vi "S4GUI.vi"(7 "Tab ObsEng":enum32{"Obs", "CCD modes", "Guider", "Eng"}(tab)) -> ()   [LabVIEW 2018] (continued)
                n2889 = call "Write Exposure Time.vi"("error in (no error)"=w6491, "Exposure Time"=w6493, "Interface in"=w6494) -> ("error out"=w6490:errorcluster, "Interface out"=w6489:refnum<class "Interface.lvclass">)  [unwired: 7 in]
              }
            }
            n2890 = case shown="True" w6212 {
              tunnel: w6214 -> [w6501 w6512]
              tunnel: [w6501 w6502] -> w6218
              tunnel: w6213 -> [w6500 w6510]
              tunnel: [w6500 w6503] -> w6217
              frame False {
              }
              frame True {
                n2891 = call-dynamic "Write restoreExpTime.vi"("error in (no error)"=w6510, "restoreExpTime"=FALSE, "Interface in"=w6512) -> ("error out"=w6509:errorcluster, "Interface out"=w6511:refnum<class "Interface.lvclass">)  [unwired: 7 in]
                n2892 = call-dynamic "Read prev ExpTime.vi"("error in (no error)"=w6509, "Interface in"=w6511) -> ("error out"=w6507:errorcluster, "prev ExpTime"=w6504:dbl, "Interface out"=w6505:refnum<class "Interface.lvclass">)  [unwired: 7 in]
                n2893 = property on="Exptime ch2" class="DigNum (strict)"(error in=w6507, "Value"=w6504) -> (error out=w6506:errorcluster)  [unwired: 1 in, 1 out]
                n2894 = call "Write Exposure Time.vi"("error in (no error)"=w6506, "Exposure Time"=w6504, "Interface in"=w6505) -> ("error out"=w6503:errorcluster, "Interface out"=w6502:refnum<class "Interface.lvclass">)  [unwired: 7 in]
              }
            }
            n2895 = case shown="True" w6265 {
              tunnel: [w6514 w6515] -> w6271
              tunnel: [w6513 w6516] -> w6270
              tunnel: w6267 -> [w6514 w6525]
              tunnel: w6266 -> [w6513 w6523]
              frame False {
              }
              frame True {
                n2896 = call-dynamic "Write restoreExpTime.vi"("error in (no error)"=w6523, "restoreExpTime"=FALSE, "Interface in"=w6525) -> ("error out"=w6522:errorcluster, "Interface out"=w6524:refnum<class "Interface.lvclass">)  [unwired: 7 in]
                n2897 = call-dynamic "Read prev ExpTime.vi"("error in (no error)"=w6522, "Interface in"=w6524) -> ("error out"=w6518:errorcluster, "prev ExpTime"=w6519:dbl, "Interface out"=w6520:refnum<class "Interface.lvclass">)  [unwired: 7 in]
                n2898 = property on="Exptime ch1" class="DigNum (strict)"(error in=w6518, "Value"=w6519) -> (error out=w6517:errorcluster)  [unwired: 1 in, 1 out]
                n2899 = call "Write Exposure Time.vi"("error in (no error)"=w6517, "Exposure Time"=w6519, "Interface in"=w6520) -> ("error out"=w6516:errorcluster, "Interface out"=w6515:refnum<class "Interface.lvclass">)  [unwired: 7 in]
              }
            }
            n2900 = call-dynamic "Read PREV_FT.vi"("error in (no error)"=w6112, "Interface in"=w6111) -> ("error out"=w6104:errorcluster, "PREV_FT"=w6113:bool, "Interface out"=w6102:refnum<class "Interface.lvclass">)  [unwired: 7 in]
            n2901 = call-dynamic "Read PREV_FT.vi"("error in (no error)"=w6217, "Interface in"=w6218) -> ("error out"=w6210:errorcluster, "PREV_FT"=w6219:bool, "Interface out"=w6208:refnum<class "Interface.lvclass">)  [unwired: 7 in]
            n2902 = call-dynamic "Read PREV_FT.vi"("error in (no error)"=w6270, "Interface in"=w6271) -> ("error out"=w6261:errorcluster, "PREV_FT"=w6272:bool, "Interface out"=w6256:refnum<class "Interface.lvclass">)  [unwired: 7 in]
            n2903 = call-dynamic "Read PREV_FT.vi"("error in (no error)"=w6164, "Interface in"=w6165) -> ("error out"=w6157:errorcluster, "PREV_FT"=w6166:bool, "Interface out"=w6155:refnum<class "Interface.lvclass">)  [unwired: 7 in]
            n2904 = call-dynamic "Read target cluster.vi"("error in (no error)"=w6104, "Channel in"=w6105) -> ("error out"=w6099:errorcluster, "target cluster"=w6103:T31, "Channel out"=w6101:refnum<class "Channel.lvclass">)  [unwired: 7 in]
            n2905 = Bundle By Name(cluster=w6103, "SHUTTER_MODE"=u8 2, "FRAME_TRANSFER"=w6113) -> (w6100:T31)
            n2906 = call-dynamic "Read target cluster.vi"("error in (no error)"=w6210, "Channel in"=w6211) -> ("error out"=w6205:errorcluster, "target cluster"=w6209:T31, "Channel out"=w6207:refnum<class "Channel.lvclass">)  [unwired: 7 in]
            n2907 = Bundle By Name(cluster=w6209, "SHUTTER_MODE"=u8 2, "FRAME_TRANSFER"=w6219) -> (w6206:T31)
            n2908 = call-dynamic "Read target cluster.vi"("error in (no error)"=w6157, "Channel in"=w6158) -> ("error out"=w6152:errorcluster, "target cluster"=w6156:T31, "Channel out"=w6154:refnum<class "Channel.lvclass">)  [unwired: 7 in]
            n2909 = Bundle By Name(cluster=w6156, "SHUTTER_MODE"=u8 2, "FRAME_TRANSFER"=w6166) -> (w6153:T31)
            n2910 = call-dynamic "Read target cluster.vi"("error in (no error)"=w6261, "Channel in"=w6264) -> ("error out"=w6260:errorcluster, "target cluster"=w6258:T31, "Channel out"=w6263:refnum<class "Channel.lvclass">)  [unwired: 7 in]
            n2911 = Bundle By Name(cluster=w6258, "SHUTTER_MODE"=u8 2, "FRAME_TRANSFER"=w6272) -> (w6257:T31)
            n2912 = call-dynamic "Write target cluster.vi"("error in (no error)"=w6260, "target cluster"=w6257, "Channel in"=w6263) -> ("error out"=w6259:errorcluster, "Channel out"=w6262:refnum<class "Channel.lvclass">)  [unwired: 7 in]
            n2913 = call-dynamic "Write target cluster.vi"("error in (no error)"=w6099, "target cluster"=w6100, "Channel in"=w6101) -> ("error out"=w6098:errorcluster, "Channel out"=w6097:refnum<class "Channel.lvclass">)  [unwired: 7 in]
            n2914 = call-dynamic "Write target cluster.vi"("error in (no error)"=w6205, "target cluster"=w6206, "Channel in"=w6207) -> ("error out"=w6204:errorcluster, "Channel out"=w6203:refnum<class "Channel.lvclass">)  [unwired: 7 in]
            n2915 = call-dynamic "Write target cluster.vi"("error in (no error)"=w6152, "target cluster"=w6153, "Channel in"=w6154) -> ("error out"=w6151:errorcluster, "Channel out"=w6150:refnum<class "Channel.lvclass">)  [unwired: 7 in]
            n2916 = Flatten To String(anything=w6257, error in (no error)=w6259) -> (data string=w6305:string, error out=w6304:errorcluster)  [unwired: 2 in, 1 out]
            n2917 = Flatten To String(anything=w6100, error in (no error)=w6098) -> (data string=w6146:string, error out=w6145:errorcluster)  [unwired: 2 in, 1 out]
            n2918 = Flatten To String(anything=w6206, error in (no error)=w6204) -> (data string=w6243:string, error out=w6244:errorcluster)  [unwired: 2 in, 1 out]
            n2919 = Flatten To String(anything=w6153, error in (no error)=w6151) -> (data string=w6190:string, error out=w6191:errorcluster)  [unwired: 2 in, 1 out]
            n2920 = call "Write flatted cluster.vi"("error in (no error)"=w6304, "flatted cluster"=w6305, "Interface in"=w6256) -> ("error out"=w6301:errorcluster, "Interface out"=w6302:refnum<class "Interface.lvclass">)  [unwired: 7 in]
            n2921 = call "Write flatted cluster.vi"("error in (no error)"=w6145, "flatted cluster"=w6146, "Interface in"=w6102) -> ("error out"=w6142:errorcluster, "Interface out"=w6143:refnum<class "Interface.lvclass">)  [unwired: 7 in]
            n2922 = call "Write flatted cluster.vi"("error in (no error)"=w6244, "flatted cluster"=w6243, "Interface in"=w6208) -> ("error out"=w6247:errorcluster, "Interface out"=w6246:refnum<class "Interface.lvclass">)  [unwired: 7 in]
            n2923 = call "Write flatted cluster.vi"("error in (no error)"=w6191, "flatted cluster"=w6190, "Interface in"=w6155) -> ("error out"=w6194:errorcluster, "Interface out"=w6193:refnum<class "Interface.lvclass">)  [unwired: 7 in]
            n2924 = call-dynamic "Write Interface.vi"("error in (no error)"=w6301, "Interface.lvclass"=w6302, "Channel in"=w6262) -> ("error out"=w6299:errorcluster, "Channel out"=w6298:refnum<class "Channel.lvclass">)  [unwired: 7 in]
            n2925 = call-dynamic "Write Interface.vi"("error in (no error)"=w6142, "Interface.lvclass"=w6143, "Channel in"=w6097) -> ("error out"=w6140:errorcluster, "Channel out"=w6139:refnum<class "Channel.lvclass">)  [unwired: 7 in]
            n2926 = call-dynamic "Write Interface.vi"("error in (no error)"=w6247, "Interface.lvclass"=w6246, "Channel in"=w6203) -> ("error out"=w6249:errorcluster, "Channel out"=w6250:refnum<class "Channel.lvclass">)  [unwired: 7 in]
            n2927 = call-dynamic "Write Interface.vi"("error in (no error)"=w6194, "Interface.lvclass"=w6193, "Channel in"=w6150) -> ("error out"=w6196:errorcluster, "Channel out"=w6197:refnum<class "Channel.lvclass">)  [unwired: 7 in]
            n2928 = call "Write section_name.vi"("error in (no error)"=w6299, "section_name"="CCD_ACS1", "Channel in"=w6298) -> ("error out"=w6300:errorcluster, "Channel out"=w6295:refnum<class "Channel.lvclass">)  [unwired: 7 in]
            n2929 = call "Write section_name.vi"("error in (no error)"=w6140, "section_name"="CCD_ACS4", "Channel in"=w6139) -> ("error out"=w6141:errorcluster, "Channel out"=w6136:refnum<class "Channel.lvclass">)  [unwired: 7 in]
            n2930 = call "Write section_name.vi"("error in (no error)"=w6249, "section_name"="CCD_ACS2", "Channel in"=w6250) -> ("error out"=w6248:errorcluster, "Channel out"=w6253:refnum<class "Channel.lvclass">)  [unwired: 7 in]
            n2931 = call "Write section_name.vi"("error in (no error)"=w6196, "section_name"="CCD_ACS3", "Channel in"=w6197) -> ("error out"=w6195:errorcluster, "Channel out"=w6200:refnum<class "Channel.lvclass">)  [unwired: 7 in]
            n2932 = call-dynamic "save config.vi"("error in (no error)"=w6300, "file config"="lastsaved.cfg", "Channel in"=w6295) -> ("error out"=w6275:errorcluster, "Channel out"=w6276:refnum<class "Channel.lvclass">)  [unwired: 7 in]
            n2933 = call-dynamic "save config.vi"("error in (no error)"=w6141, "file config"="lastsaved.cfg", "Channel in"=w6136) -> ("error out"=w6116:errorcluster, "Channel out"=w6117:refnum<class "Channel.lvclass">)  [unwired: 7 in]
            n2934 = call-dynamic "save config.vi"("error in (no error)"=w6248, "file config"="lastsaved.cfg", "Channel in"=w6253) -> ("error out"=w6222:errorcluster, "Channel out"=w6223:refnum<class "Channel.lvclass">)  [unwired: 7 in]
            n2935 = call-dynamic "save config.vi"("error in (no error)"=w6195, "file config"="lastsaved.cfg", "Channel in"=w6200) -> ("error out"=w6169:errorcluster, "Channel out"=w6170:refnum<class "Channel.lvclass">)  [unwired: 7 in]
            n2936 = local read "Filter1"() -> (w6277:u8)
            n2937 = local read "Filter2"() -> (w6224:u8)
            n2938 = local read "Filter4"() -> (w6118:u8)
            n2939 = local read "Filter3"() -> (w6171:u8)
            n2940 = call-dynamic "Write Filter.vi"("error in (no error)"=w6275, "Filter"=w6277, "Channel in"=w6276) -> ("error out"=w6284:errorcluster, "Channel out"=w6285:refnum<class "Channel.lvclass">)  [unwired: 7 in]
            n2941 = call-dynamic "Write Filter.vi"("error in (no error)"=w6169, "Filter"=w6171, "Channel in"=w6170) -> ("error out"=w6178:errorcluster, "Channel out"=w6179:refnum<class "Channel.lvclass">)  [unwired: 7 in]
            n2942 = call-dynamic "Write Filter.vi"("error in (no error)"=w6222, "Filter"=w6224, "Channel in"=w6223) -> ("error out"=w6231:errorcluster, "Channel out"=w6232:refnum<class "Channel.lvclass">)  [unwired: 7 in]
            n2943 = call-dynamic "Write Filter.vi"("error in (no error)"=w6116, "Filter"=w6118, "Channel in"=w6117) -> ("error out"=w6125:errorcluster, "Channel out"=w6126:refnum<class "Channel.lvclass">)  [unwired: 7 in]
            n2944 = call-dynamic "Read Interface.vi"("error in (no error)"=w6231, "Channel in"=w6232) -> ("error out"=w6229:errorcluster, "Interface.lvclass"=w6234:refnum<class "Interface.lvclass">, "Channel out"=w6233:refnum<class "Channel.lvclass">)  [unwired: 7 in]
            n2945 = call-dynamic "Read Interface.vi"("error in (no error)"=w6178, "Channel in"=w6179) -> ("error out"=w6176:errorcluster, "Interface.lvclass"=w6181:refnum<class "Interface.lvclass">, "Channel out"=w6180:refnum<class "Channel.lvclass">)  [unwired: 7 in]
            n2946 = call-dynamic "Read Interface.vi"("error in (no error)"=w6284, "Channel in"=w6285) -> ("error out"=w6282:errorcluster, "Interface.lvclass"=w6287:refnum<class "Interface.lvclass">, "Channel out"=w6286:refnum<class "Channel.lvclass">)  [unwired: 7 in]
            n2947 = call-dynamic "Read Interface.vi"("error in (no error)"=w6125, "Channel in"=w6126) -> ("error out"=w6123:errorcluster, "Interface.lvclass"=w6128:refnum<class "Interface.lvclass">, "Channel out"=w6127:refnum<class "Channel.lvclass">)  [unwired: 7 in]
            n2948 = call-dynamic "Write Suffix.vi"("error in (no error)"=w6282, "Suffix"=w6310, "Interface in"=w6287) -> ("error out"=w6278:errorcluster, "Interface out"=w6288:refnum<class "Interface.lvclass">)  [unwired: 7 in]
            n2949 = call-dynamic "Write Suffix.vi"("error in (no error)"=w6229, "Suffix"=w6310, "Interface in"=w6234) -> ("error out"=w6225:errorcluster, "Interface out"=w6235:refnum<class "Interface.lvclass">)  [unwired: 7 in]
            n2950 = call-dynamic "Write Suffix.vi"("error in (no error)"=w6176, "Suffix"=w6310, "Interface in"=w6181) -> ("error out"=w6172:errorcluster, "Interface out"=w6182:refnum<class "Interface.lvclass">)  [unwired: 7 in]
            n2951 = call-dynamic "Write Suffix.vi"("error in (no error)"=w6123, "Suffix"=w6310, "Interface in"=w6128) -> ("error out"=w6119:errorcluster, "Interface out"=w6129:refnum<class "Interface.lvclass">)  [unwired: 7 in]
            n2952 = call-dynamic "Write ObsType.vi"("error in (no error)"=w6225, "ObsType"=w6309, "Interface in"=w6235) -> ("error out"=w6226:errorcluster, "Interface out"=w6236:refnum<class "Interface.lvclass">)  [unwired: 7 in]
            n2953 = call-dynamic "Write ObsType.vi"("error in (no error)"=w6172, "ObsType"=w6309, "Interface in"=w6182) -> ("error out"=w6173:errorcluster, "Interface out"=w6183:refnum<class "Interface.lvclass">)  [unwired: 7 in]
            n2954 = call-dynamic "Write ObsType.vi"("error in (no error)"=w6278, "ObsType"=w6309, "Interface in"=w6288) -> ("error out"=w6279:errorcluster, "Interface out"=w6289:refnum<class "Interface.lvclass">)  [unwired: 7 in]
            n2955 = call-dynamic "Write ObsType.vi"("error in (no error)"=w6119, "ObsType"=w6309, "Interface in"=w6129) -> ("error out"=w6120:errorcluster, "Interface out"=w6130:refnum<class "Interface.lvclass">)  [unwired: 7 in]
            n2956 = call-dynamic "Write Object.vi"("error in (no error)"=w6226, "Object"=w6313, "Interface in"=w6236) -> ("error out"=w6227:errorcluster, "Interface out"=w6237:refnum<class "Interface.lvclass">)  [unwired: 7 in]
            n2957 = call-dynamic "Write Object.vi"("error in (no error)"=w6173, "Object"=w6313, "Interface in"=w6183) -> ("error out"=w6174:errorcluster, "Interface out"=w6184:refnum<class "Interface.lvclass">)  [unwired: 7 in]
            n2958 = call-dynamic "Write Object.vi"("error in (no error)"=w6279, "Object"=w6313, "Interface in"=w6289) -> ("error out"=w6280:errorcluster, "Interface out"=w6290:refnum<class "Interface.lvclass">)  [unwired: 7 in]
            n2959 = call-dynamic "Write Object.vi"("error in (no error)"=w6120, "Object"=w6313, "Interface in"=w6130) -> ("error out"=w6121:errorcluster, "Interface out"=w6131:refnum<class "Interface.lvclass">)  [unwired: 7 in]
            n2960 = call-dynamic "Write Comments.vi"("error in (no error)"=w6227, "Comments"=w6312, "Interface in"=w6237) -> ("error out"=w6228:errorcluster, "Interface out"=w6238:refnum<class "Interface.lvclass">)  [unwired: 7 in]
            n2961 = call-dynamic "Write Comments.vi"("error in (no error)"=w6174, "Comments"=w6312, "Interface in"=w6184) -> ("error out"=w6175:errorcluster, "Interface out"=w6185:refnum<class "Interface.lvclass">)  [unwired: 7 in]
            n2962 = call-dynamic "Write Comments.vi"("error in (no error)"=w6280, "Comments"=w6312, "Interface in"=w6290) -> ("error out"=w6281:errorcluster, "Interface out"=w6291:refnum<class "Interface.lvclass">)  [unwired: 7 in]
            n2963 = call-dynamic "Write Comments.vi"("error in (no error)"=w6121, "Comments"=w6312, "Interface in"=w6131) -> ("error out"=w6122:errorcluster, "Interface out"=w6132:refnum<class "Interface.lvclass">)  [unwired: 7 in]
            n2964 = call-dynamic "Write Observer.vi"("error in (no error)"=w6228, "Observer"=w6311, "Interface in"=w6238) -> ("error out"=w6230:errorcluster, "Interface out"=w6239:refnum<class "Interface.lvclass">)  [unwired: 7 in]
            n2965 = call-dynamic "Write Observer.vi"("error in (no error)"=w6175, "Observer"=w6311, "Interface in"=w6185) -> ("error out"=w6177:errorcluster, "Interface out"=w6186:refnum<class "Interface.lvclass">)  [unwired: 7 in]
            n2966 = call-dynamic "Write Observer.vi"("error in (no error)"=w6281, "Observer"=w6311, "Interface in"=w6291) -> ("error out"=w6283:errorcluster, "Interface out"=w6292:refnum<class "Interface.lvclass">)  [unwired: 7 in]
            n2967 = call-dynamic "Write Observer.vi"("error in (no error)"=w6122, "Observer"=w6311, "Interface in"=w6132) -> ("error out"=w6124:errorcluster, "Interface out"=w6133:refnum<class "Interface.lvclass">)  [unwired: 7 in]
            n2968 = call-dynamic "Write Interface.vi"("error in (no error)"=w6230, "Interface.lvclass"=w6239, "Channel in"=w6233) -> ("error out"=w6220:errorcluster, "Channel out"=w6221:refnum<class "Channel.lvclass">)  [unwired: 7 in]
            n2969 = call-dynamic "Write Interface.vi"("error in (no error)"=w6177, "Interface.lvclass"=w6186, "Channel in"=w6180) -> ("error out"=w6167:errorcluster, "Channel out"=w6168:refnum<class "Channel.lvclass">)  [unwired: 7 in]
            n2970 = call-dynamic "Write Interface.vi"("error in (no error)"=w6283, "Interface.lvclass"=w6292, "Channel in"=w6286) -> ("error out"=w6273:errorcluster, "Channel out"=w6274:refnum<class "Channel.lvclass">)  [unwired: 7 in]
            n2971 = call-dynamic "Write Interface.vi"("error in (no error)"=w6124, "Interface.lvclass"=w6133, "Channel in"=w6127) -> ("error out"=w6114:errorcluster, "Channel out"=w6115:refnum<class "Channel.lvclass">)  [unwired: 7 in]
            n2972 = case shown="True" w6096 {
              tunnel: [w6441 w6462] -> w6294
              tunnel: [w6440 w6461] -> w6293
              tunnel: w6274 -> [w6441 w6460]
              tunnel: w6273 -> [w6440 w6459]
              frame False {
              }
              frame True {
                # "command SET EXPTIME"
                # "command WRITE_SETUP"
                # "command SET SUFFIX"
                n2973 = call-dynamic "Read State Machine.vi"("error in (no error)"=w6459, "Device in"=w6460) -> ("error out"=w6449:errorcluster, "State Machine.lvclass"=w6451:refnum<class "State Machine.lvclass">, "Device out"=w6464:refnum<class "Channel.lvclass">)  [unwired: 7 in]
                n2974 = call-dynamic "Read ref StatesQueue.vi"("error in (no error)"=w6449, "State Machine in"=w6451) -> ("error out"=w6457:errorcluster, "ref StatesQueue"=w6447:refnum<queue>, "State Machine out"=w6458:refnum<class "State Machine.lvclass">)  [unwired: 7 in]
                n2975 = Flush Queue(queue=w6447, error in (no error)=w6457) -> (queue out=w6446:refnum<queue>, error out=w6454:errorcluster)  [unwired: 1 out]
                n2976 = Enqueue Element(queue=w6446, element=u32 300 ("State"), error in (no error)=w6454) -> (queue out=w6445:refnum<queue>, error out=w6444:errorcluster)  [unwired: 1 in, 1 out]
                n2977 = disable-structure shown="Enabled" {
                  disable-tunnel: w6445 -> [w6470 w6473]
                  disable-tunnel: w6444 -> [w6469 w6472]
                  disable-tunnel: [w6468 w6472] -> w6443
                  disable-tunnel: [w6467 w6473] -> w6442
                  frame Disabled {
                    n2978 = Enqueue Element(queue=w6470, element=u32 305 ("State"), error in (no error)=w6469) -> (queue out=w6467:refnum<queue>, error out=w6468:errorcluster)  [unwired: 1 in, 1 out]
                  }
                  frame Enabled {
                  }
                }
                n2979 = Enqueue Element(queue=w6442, element=u32 60 ("State"), error in (no error)=w6443) -> (queue out=w6456:refnum<queue>, error out=w6455:errorcluster)  [unwired: 1 in, 1 out]
                n2980 = call-dynamic "Write ref StatesQueue.vi"("error in (no error)"=w6455, "ref StatesQueue"=w6456, "State Machine in"=w6458) -> ("error out"=w6448:errorcluster, "State Machine out"=w6450:refnum<class "State Machine.lvclass">)  [unwired: 7 in]
                n2981 = call-dynamic "Write State.vi"("error in (no error)"=w6448, "State"=0, "State Machine in"=w6450) -> ("error out"=w6466:errorcluster, "State Machine out"=w6463:refnum<class "State Machine.lvclass">)  [unwired: 7 in]
                n2982 = call-dynamic "Write State Machine.vi"("error in (no error)"=w6466, "State Machine.lvclass"=w6463, "Device in"=w6464) -> ("error out"=w6461:errorcluster, "Device out"=w6462:refnum<class "Channel.lvclass">)  [unwired: 7 in]
              }
            }
            n2983 = case shown="True" w6095 {
              tunnel: [w6406 w6432] -> w6255
              tunnel: [w6407 w6431] -> w6254
              tunnel: w6221 -> [w6407 w6426]
              tunnel: w6220 -> [w6406 w6425]
              frame False {
              }
              frame True {
                # "command SET EXPTIME"
                # "command WRITE_SETUP"
                # "command SET SUFFIX"
                n2984 = call-dynamic "Read State Machine.vi"("error in (no error)"=w6425, "Device in"=w6426) -> ("error out"=w6416:errorcluster, "State Machine.lvclass"=w6417:refnum<class "State Machine.lvclass">, "Device out"=w6429:refnum<class "Channel.lvclass">)  [unwired: 7 in]
                n2985 = call-dynamic "Read ref StatesQueue.vi"("error in (no error)"=w6416, "State Machine in"=w6417) -> ("error out"=w6423:errorcluster, "ref StatesQueue"=w6415:refnum<queue>, "State Machine out"=w6424:refnum<class "State Machine.lvclass">)  [unwired: 7 in]
                n2986 = Flush Queue(queue=w6415, error in (no error)=w6423) -> (queue out=w6414:refnum<queue>, error out=w6420:errorcluster)  [unwired: 1 out]
                n2987 = Enqueue Element(queue=w6414, element=u32 300 ("State"), error in (no error)=w6420) -> (queue out=w6409:refnum<queue>, error out=w6411:errorcluster)  [unwired: 1 in, 1 out]
                n2988 = disable-structure shown="Enabled" {
                  disable-tunnel: w6411 -> [w6436 w6438]
                  disable-tunnel: [w6435 w6438] -> w6410
                  disable-tunnel: w6409 -> [w6434 w6439]
                  disable-tunnel: [w6433 w6439] -> w6408
                  frame Disabled {
                    n2989 = Enqueue Element(queue=w6434, element=u32 305 ("State"), error in (no error)=w6436) -> (queue out=w6433:refnum<queue>, error out=w6435:errorcluster)  [unwired: 1 in, 1 out]
                  }
                  frame Enabled {
                  }
                }
                n2990 = Enqueue Element(queue=w6408, element=u32 60 ("State"), error in (no error)=w6410) -> (queue out=w6422:refnum<queue>, error out=w6421:errorcluster)  [unwired: 1 in, 1 out]
                n2991 = call-dynamic "Write ref StatesQueue.vi"("error in (no error)"=w6421, "ref StatesQueue"=w6422, "State Machine in"=w6424) -> ("error out"=w6412:errorcluster, "State Machine out"=w6413:refnum<class "State Machine.lvclass">)  [unwired: 7 in]
                n2992 = call-dynamic "Write State.vi"("error in (no error)"=w6412, "State"=0, "State Machine in"=w6413) -> ("error out"=w6427:errorcluster, "State Machine out"=w6430:refnum<class "State Machine.lvclass">)  [unwired: 7 in]
                n2993 = call-dynamic "Write State Machine.vi"("error in (no error)"=w6427, "State Machine.lvclass"=w6430, "Device in"=w6429) -> ("error out"=w6432:errorcluster, "Device out"=w6431:refnum<class "Channel.lvclass">)  [unwired: 7 in]
              }
            }
            n2994 = case shown="True" w6094 {
              tunnel: [w6372 w6398] -> w6202
              tunnel: [w6373 w6397] -> w6201
              tunnel: w6168 -> [w6373 w6392]
              tunnel: w6167 -> [w6372 w6391]
              frame False {
              }
              frame True {
                # "command SET EXPTIME"
                # "command WRITE_SETUP"
                # "command SET SUFFIX"
                n2995 = call-dynamic "Read State Machine.vi"("error in (no error)"=w6391, "Device in"=w6392) -> ("error out"=w6381:errorcluster, "State Machine.lvclass"=w6380:refnum<class "State Machine.lvclass">, "Device out"=w6395:refnum<class "Channel.lvclass">)  [unwired: 7 in]
                n2996 = call-dynamic "Read ref StatesQueue.vi"("error in (no error)"=w6381, "State Machine in"=w6380) -> ("error out"=w6389:errorcluster, "ref StatesQueue"=w6383:refnum<queue>, "State Machine out"=w6390:refnum<class "State Machine.lvclass">)  [unwired: 7 in]
                n2997 = Flush Queue(queue=w6383, error in (no error)=w6389) -> (queue out=w6382:refnum<queue>, error out=w6386:errorcluster)  [unwired: 1 out]
                n2998 = Enqueue Element(queue=w6382, element=u32 300 ("State"), error in (no error)=w6386) -> (queue out=w6376:refnum<queue>, error out=w6377:errorcluster)  [unwired: 1 in, 1 out]
                n2999 = disable-structure shown="Enabled" {
                  disable-tunnel: w6377 -> [w6402 w6404]
                  disable-tunnel: w6376 -> [w6401 w6405]
                  disable-tunnel: [w6400 w6404] -> w6375
                  disable-tunnel: [w6399 w6405] -> w6374
                  frame Disabled {
                    n3000 = Enqueue Element(queue=w6401, element=u32 305 ("State"), error in (no error)=w6402) -> (queue out=w6399:refnum<queue>, error out=w6400:errorcluster)  [unwired: 1 in, 1 out]
                  }
                  frame Enabled {
                  }
                }
                n3001 = Enqueue Element(queue=w6374, element=u32 60 ("State"), error in (no error)=w6375) -> (queue out=w6388:refnum<queue>, error out=w6387:errorcluster)  [unwired: 1 in, 1 out]
                n3002 = call-dynamic "Write ref StatesQueue.vi"("error in (no error)"=w6387, "ref StatesQueue"=w6388, "State Machine in"=w6390) -> ("error out"=w6378:errorcluster, "State Machine out"=w6379:refnum<class "State Machine.lvclass">)  [unwired: 7 in]
                n3003 = call-dynamic "Write State.vi"("error in (no error)"=w6378, "State"=0, "State Machine in"=w6379) -> ("error out"=w6393:errorcluster, "State Machine out"=w6396:refnum<class "State Machine.lvclass">)  [unwired: 7 in]
                n3004 = call-dynamic "Write State Machine.vi"("error in (no error)"=w6393, "State Machine.lvclass"=w6396, "Device in"=w6395) -> ("error out"=w6398:errorcluster, "Device out"=w6397:refnum<class "Channel.lvclass">)  [unwired: 7 in]
              }
            }
            n3005 = case shown="True" w6093 {
              tunnel: [w6338 w6360] -> w6135
              tunnel: [w6339 w6359] -> w6134
              tunnel: w6115 -> [w6339 w6358]
              tunnel: w6114 -> [w6338 w6357]
              frame False {
              }
              frame True {
                # "command SET EXPTIME"
                # "command WRITE_SETUP"
                # "command SET SUFFIX"
                n3006 = call-dynamic "Read State Machine.vi"("error in (no error)"=w6357, "Device in"=w6358) -> ("error out"=w6346:errorcluster, "State Machine.lvclass"=w6347:refnum<class "State Machine.lvclass">, "Device out"=w6362:refnum<class "Channel.lvclass">)  [unwired: 7 in]
                n3007 = call-dynamic "Read ref StatesQueue.vi"("error in (no error)"=w6346, "State Machine in"=w6347) -> ("error out"=w6355:errorcluster, "ref StatesQueue"=w6349:refnum<queue>, "State Machine out"=w6356:refnum<class "State Machine.lvclass">)  [unwired: 7 in]
                n3008 = Flush Queue(queue=w6349, error in (no error)=w6355) -> (queue out=w6348:refnum<queue>, error out=w6352:errorcluster)  [unwired: 1 out]
                n3009 = Enqueue Element(queue=w6348, element=u32 300 ("State"), error in (no error)=w6352) -> (queue out=w6343:refnum<queue>, error out=w6341:errorcluster)  [unwired: 1 in, 1 out]
                n3010 = disable-structure shown="Enabled" {
                  disable-tunnel: w6343 -> [w6368 w6371]
                  disable-tunnel: [w6367 w6371] -> w6342
                  disable-tunnel: w6341 -> [w6366 w6370]
                  disable-tunnel: [w6365 w6370] -> w6340
                  frame Disabled {
                    n3011 = Enqueue Element(queue=w6368, element=u32 305 ("State"), error in (no error)=w6366) -> (queue out=w6367:refnum<queue>, error out=w6365:errorcluster)  [unwired: 1 in, 1 out]
                  }
                  frame Enabled {
                  }
                }
                n3012 = Enqueue Element(queue=w6342, element=u32 60 ("State"), error in (no error)=w6340) -> (queue out=w6354:refnum<queue>, error out=w6353:errorcluster)  [unwired: 1 in, 1 out]
                n3013 = call-dynamic "Write ref StatesQueue.vi"("error in (no error)"=w6353, "ref StatesQueue"=w6354, "State Machine in"=w6356) -> ("error out"=w6344:errorcluster, "State Machine out"=w6345:refnum<class "State Machine.lvclass">)  [unwired: 7 in]
                n3014 = call-dynamic "Write State.vi"("error in (no error)"=w6344, "State"=0, "State Machine in"=w6345) -> ("error out"=w6364:errorcluster, "State Machine out"=w6361:refnum<class "State Machine.lvclass">)  [unwired: 7 in]
                n3015 = call-dynamic "Write State Machine.vi"("error in (no error)"=w6364, "State Machine.lvclass"=w6361, "Device in"=w6362) -> ("error out"=w6360:errorcluster, "Device out"=w6359:refnum<class "Channel.lvclass">)  [unwired: 7 in]
              }
            }
            n3016 = call-dynamic "Write Channel.vi"("error in (no error)"=w6255, "Channel.lvclass"=w6254, "Acquisition in"=w6240) -> ("error out"=w6334:errorcluster, "Acquisition out"=w6335:refnum<class "Acquisition.lvclass">)  [unwired: 7 in]
            n3017 = call-dynamic "Write Channel.vi"("error in (no error)"=w6135, "Channel.lvclass"=w6134, "Acquisition in"=w6149) -> ("error out"=w6330:errorcluster, "Acquisition out"=w6331:refnum<class "Acquisition.lvclass">)  [unwired: 7 in]
            n3018 = call-dynamic "Write Channel.vi"("error in (no error)"=w6293, "Channel.lvclass"=w6294, "Acquisition in"=w6308) -> ("error out"=w6336:errorcluster, "Acquisition out"=w6337:refnum<class "Acquisition.lvclass">)  [unwired: 7 in]
            n3019 = call-dynamic "Write Channel.vi"("error in (no error)"=w6202, "Channel.lvclass"=w6201, "Acquisition in"=w6187) -> ("error out"=w6332:errorcluster, "Acquisition out"=w6333:refnum<class "Acquisition.lvclass">)  [unwired: 7 in]
          }
          frame "OBJECT", Default {
            # "20250918:\nACS corrigido,\nnão precisa restaurar\nExpTime. Causou bug\nquando ExpTime tinha\nvalor default (1E-5s)"
            # "nome do arquivo .cfg"
            # "seção no arquivo .cfg"
            # "open"
            # "nome do arquivo .cfg"
            # "seção no arquivo .cfg"
            # "open"
            # "nome do arquivo .cfg"
            # "seção no arquivo .cfg"
            # "open"
            # "nome do arquivo .cfg"
            # "seção no arquivo .cfg"
            # "open"
            # "OBJECT, DFLAT,SFLAT and FOCUS: Shutter automatically open and restore FRAME_TRANSFER."
            n3020 = call "Read connection.vi"("error in (no error)"=w6751, "Server in"=w6752) -> ("error out"=w6757:errorcluster, "connection"=w6527:bool, "Server out"=w6758:refnum<class "Acquisition.lvclass">)  [unwired: 7 in]
            n3021 = call "Read connection.vi"("error in (no error)"=w6749, "Server in"=w6750) -> ("error out"=w6755:errorcluster, "connection"=w6528:bool, "Server out"=w6756:refnum<class "Acquisition.lvclass">)  [unwired: 7 in]
            n3022 = call "Read connection.vi"("error in (no error)"=w6761, "Server in"=w6762) -> ("error out"=w6759:errorcluster, "connection"=w6526:bool, "Server out"=w6760:refnum<class "Acquisition.lvclass">)  [unwired: 7 in]
            n3023 = call "Read connection.vi"("error in (no error)"=w6747, "Server in"=w6748) -> ("error out"=w6753:errorcluster, "connection"=w6529:bool, "Server out"=w6754:refnum<class "Acquisition.lvclass">)  [unwired: 7 in]
            n3024 = call-dynamic "Read Channel.vi"("error in (no error)"=w6753, "Acquisition in"=w6754) -> ("error out"=w6580:errorcluster, "Channel.lvclass"=w6581:refnum<class "Channel.lvclass">, "Acquisition out"=w6582:refnum<class "Acquisition.lvclass">)  [unwired: 7 in]
            n3025 = call-dynamic "Read Channel.vi"("error in (no error)"=w6759, "Acquisition in"=w6760) -> ("error out"=w6739:errorcluster, "Channel.lvclass"=w6740:refnum<class "Channel.lvclass">, "Acquisition out"=w6741:refnum<class "Acquisition.lvclass">)  [unwired: 7 in]
            n3026 = call-dynamic "Read Channel.vi"("error in (no error)"=w6755, "Acquisition in"=w6756) -> ("error out"=w6624:errorcluster, "Channel.lvclass"=w6623:refnum<class "Channel.lvclass">, "Acquisition out"=w6622:refnum<class "Acquisition.lvclass">)  [unwired: 7 in]
            n3027 = call-dynamic "Read Channel.vi"("error in (no error)"=w6757, "Acquisition in"=w6758) -> ("error out"=w6677:errorcluster, "Channel.lvclass"=w6676:refnum<class "Channel.lvclass">, "Acquisition out"=w6675:refnum<class "Acquisition.lvclass">)  [unwired: 7 in]
            n3028 = call-dynamic "Read Interface.vi"("error in (no error)"=w6580, "Channel in"=w6581) -> ("error out"=w6548:errorcluster, "Interface.lvclass"=w6549:refnum<class "Interface.lvclass">, "Channel out"=w6545:refnum<class "Channel.lvclass">)  [unwired: 7 in]
            n3029 = call-dynamic "Read Interface.vi"("error in (no error)"=w6739, "Channel in"=w6740) -> ("error out"=w6701:errorcluster, "Interface.lvclass"=w6702:refnum<class "Interface.lvclass">, "Channel out"=w6691:refnum<class "Channel.lvclass">)  [unwired: 7 in]
            n3030 = call-dynamic "Read Interface.vi"("error in (no error)"=w6624, "Channel in"=w6623) -> ("error out"=w6598:errorcluster, "Interface.lvclass"=w6600:refnum<class "Interface.lvclass">, "Channel out"=w6595:refnum<class "Channel.lvclass">)  [unwired: 7 in]
            n3031 = call-dynamic "Read Interface.vi"("error in (no error)"=w6677, "Channel in"=w6676) -> ("error out"=w6651:errorcluster, "Interface.lvclass"=w6653:refnum<class "Interface.lvclass">, "Channel out"=w6648:refnum<class "Channel.lvclass">)  [unwired: 7 in]
            n3032 = call-dynamic "Read restoreExpTime.vi"("error in (no error)"=w6548, "Interface in"=w6549) -> ("error out"=w6547:errorcluster, "restoreExpTime"=w6550:bool, "Interface out"=w6546:refnum<class "Interface.lvclass">)  [unwired: 7 in]
            n3033 = call-dynamic "Read restoreExpTime.vi"("error in (no error)"=w6701, "Interface in"=w6702) -> ("error out"=w6699:errorcluster, "restoreExpTime"=w6698:bool, "Interface out"=w6700:refnum<class "Interface.lvclass">)  [unwired: 7 in]
            n3034 = call-dynamic "Read restoreExpTime.vi"("error in (no error)"=w6651, "Interface in"=w6653) -> ("error out"=w6650:errorcluster, "restoreExpTime"=w6649:bool, "Interface out"=w6652:refnum<class "Interface.lvclass">)  [unwired: 7 in]
            n3035 = call-dynamic "Read restoreExpTime.vi"("error in (no error)"=w6598, "Interface in"=w6600) -> ("error out"=w6597:errorcluster, "restoreExpTime"=w6596:bool, "Interface out"=w6599:refnum<class "Interface.lvclass">)  [unwired: 7 in]
            n3036 = case shown="True" w6550 {
              tunnel: w6546 -> [w6908 w6919]
              tunnel: [w6908 w6910] -> w6552
              tunnel: w6547 -> [w6907 w6918]
              tunnel: [w6907 w6909] -> w6551
              frame False {
              }
              frame True {
                n3037 = call-dynamic "Write restoreExpTime.vi"("error in (no error)"=w6918, "restoreExpTime"=FALSE, "Interface in"=w6919) -> ("error out"=w6916:errorcluster, "Interface out"=w6917:refnum<class "Interface.lvclass">)  [unwired: 7 in]
                n3038 = call-dynamic "Read prev ExpTime.vi"("error in (no error)"=w6916, "Interface in"=w6917) -> ("error out"=w6911:errorcluster, "prev ExpTime"=w6913:dbl, "Interface out"=w6914:refnum<class "Interface.lvclass">)  [unwired: 7 in]
                n3039 = property on="Exptime ch4" class="DigNum (strict)"(error in=w6911, "Value"=w6913) -> (error out=w6912:errorcluster)  [unwired: 1 in, 1 out]
                n3040 = call "Write Exposure Time.vi"("error in (no error)"=w6912, "Exposure Time"=w6913, "Interface in"=w6914) -> ("error out"=w6909:errorcluster, "Interface out"=w6910:refnum<class "Interface.lvclass">)  [unwired: 7 in]
              }
            }
            n3041 = case shown="True" w6698 {
              tunnel: w6700 -> [w6947 w6958]
              tunnel: [w6947 w6951] -> w6704
              tunnel: w6699 -> [w6946 w6956]
              tunnel: [w6946 w6952] -> w6703
              frame False {
              }
              frame True {
                n3042 = call-dynamic "Write restoreExpTime.vi"("error in (no error)"=w6956, "restoreExpTime"=FALSE, "Interface in"=w6958) -> ("error out"=w6955:errorcluster, "Interface out"=w6957:refnum<class "Interface.lvclass">)  [unwired: 7 in]
                n3043 = call-dynamic "Read prev ExpTime.vi"("error in (no error)"=w6955, "Interface in"=w6957) -> ("error out"=w6949:errorcluster, "prev ExpTime"=w6950:dbl, "Interface out"=w6953:refnum<class "Interface.lvclass">)  [unwired: 7 in]
                n3044 = property on="Exptime ch1" class="DigNum (strict)"(error in=w6949, "Value"=w6950) -> (error out=w6948:errorcluster)  [unwired: 1 in, 1 out]
                n3045 = call "Write Exposure Time.vi"("error in (no error)"=w6948, "Exposure Time"=w6950, "Interface in"=w6953) -> ("error out"=w6952:errorcluster, "Interface out"=w6951:refnum<class "Interface.lvclass">)  [unwired: 7 in]
              }
            }
            n3046 = case shown="True" w6596 {
              tunnel: w6599 -> [w6921 w6932]
              tunnel: [w6921 w6922] -> w6602
              tunnel: w6597 -> [w6920 w6931]
              tunnel: [w6920 w6923] -> w6601
              frame False {
              }
              frame True {
                n3047 = call-dynamic "Write restoreExpTime.vi"("error in (no error)"=w6931, "restoreExpTime"=FALSE, "Interface in"=w6932) -> ("error out"=w6929:errorcluster, "Interface out"=w6930:refnum<class "Interface.lvclass">)  [unwired: 7 in]
                n3048 = call-dynamic "Read prev ExpTime.vi"("error in (no error)"=w6929, "Interface in"=w6930) -> ("error out"=w6925:errorcluster, "prev ExpTime"=w6926:dbl, "Interface out"=w6927:refnum<class "Interface.lvclass">)  [unwired: 7 in]
                n3049 = property on="Exptime ch3" class="DigNum (strict)"(error in=w6925, "Value"=w6926) -> (error out=w6924:errorcluster)  [unwired: 1 in, 1 out]
                n3050 = call "Write Exposure Time.vi"("error in (no error)"=w6924, "Exposure Time"=w6926, "Interface in"=w6927) -> ("error out"=w6923:errorcluster, "Interface out"=w6922:refnum<class "Interface.lvclass">)  [unwired: 7 in]
              }
            }
            n3051 = case shown="True" w6649 {
              tunnel: w6652 -> [w6934 w6945]
              tunnel: [w6934 w6939] -> w6655
              tunnel: w6650 -> [w6933 w6944]
              tunnel: [w6933 w6935] -> w6654
              frame False {
              }
              frame True {
                n3052 = call-dynamic "Write restoreExpTime.vi"("error in (no error)"=w6944, "restoreExpTime"=FALSE, "Interface in"=w6945) -> ("error out"=w6942:errorcluster, "Interface out"=w6943:refnum<class "Interface.lvclass">)  [unwired: 7 in]
                n3053 = call-dynamic "Read prev ExpTime.vi"("error in (no error)"=w6942, "Interface in"=w6943) -> ("error out"=w6938:errorcluster, "prev ExpTime"=w6937:dbl, "Interface out"=w6940:refnum<class "Interface.lvclass">)  [unwired: 7 in]
                n3054 = property on="Exptime ch2" class="DigNum (strict)"(error in=w6938, "Value"=w6937) -> (error out=w6936:errorcluster)  [unwired: 1 in, 1 out]
                n3055 = call "Write Exposure Time.vi"("error in (no error)"=w6936, "Exposure Time"=w6937, "Interface in"=w6940) -> ("error out"=w6935:errorcluster, "Interface out"=w6939:refnum<class "Interface.lvclass">)  [unwired: 7 in]
              }
            }
            n3056 = call-dynamic "Read PREV_FT.vi"("error in (no error)"=w6551, "Interface in"=w6552) -> ("error out"=w6544:errorcluster, "PREV_FT"=w6553:bool, "Interface out"=w6542:refnum<class "Interface.lvclass">)  [unwired: 7 in]
            n3057 = call-dynamic "Read PREV_FT.vi"("error in (no error)"=w6654, "Interface in"=w6655) -> ("error out"=w6646:errorcluster, "PREV_FT"=w6656:bool, "Interface out"=w6645:refnum<class "Interface.lvclass">)  [unwired: 7 in]
            n3058 = call-dynamic "Read PREV_FT.vi"("error in (no error)"=w6601, "Interface in"=w6602) -> ("error out"=w6593:errorcluster, "PREV_FT"=w6603:bool, "Interface out"=w6592:refnum<class "Interface.lvclass">)  [unwired: 7 in]
            n3059 = call-dynamic "Read PREV_FT.vi"("error in (no error)"=w6703, "Interface in"=w6704) -> ("error out"=w6697:errorcluster, "PREV_FT"=w6705:bool, "Interface out"=w6696:refnum<class "Interface.lvclass">)  [unwired: 7 in]
            n3060 = call-dynamic "Read target cluster.vi"("error in (no error)"=w6544, "Channel in"=w6545) -> ("error out"=w6539:errorcluster, "target cluster"=w6543:T31, "Channel out"=w6541:refnum<class "Channel.lvclass">)  [unwired: 7 in]
            n3061 = Bundle By Name(cluster=w6543, "SHUTTER_MODE"=u8 1, "FRAME_TRANSFER"=w6553) -> (w6540:T31)
            n3062 = call-dynamic "Read target cluster.vi"("error in (no error)"=w6697, "Channel in"=w6691) -> ("error out"=w6692:errorcluster, "target cluster"=w6695:T31, "Channel out"=w6690:refnum<class "Channel.lvclass">)  [unwired: 7 in]
            n3063 = Bundle By Name(cluster=w6695, "SHUTTER_MODE"=u8 1, "FRAME_TRANSFER"=w6705) -> (w6694:T31)
            n3064 = call-dynamic "Read target cluster.vi"("error in (no error)"=w6646, "Channel in"=w6648) -> ("error out"=w6643:errorcluster, "target cluster"=w6647:T31, "Channel out"=w6641:refnum<class "Channel.lvclass">)  [unwired: 7 in]
            n3065 = Bundle By Name(cluster=w6647, "SHUTTER_MODE"=u8 1, "FRAME_TRANSFER"=w6656) -> (w6644:T31)
            n3066 = call-dynamic "Read target cluster.vi"("error in (no error)"=w6593, "Channel in"=w6595) -> ("error out"=w6590:errorcluster, "target cluster"=w6594:T31, "Channel out"=w6588:refnum<class "Channel.lvclass">)  [unwired: 7 in]
            n3067 = Bundle By Name(cluster=w6594, "SHUTTER_MODE"=u8 1, "FRAME_TRANSFER"=w6603) -> (w6591:T31)
            n3068 = call-dynamic "Write target cluster.vi"("error in (no error)"=w6539, "target cluster"=w6540, "Channel in"=w6541) -> ("error out"=w6538:errorcluster, "Channel out"=w6537:refnum<class "Channel.lvclass">)  [unwired: 7 in]
            n3069 = call-dynamic "Write target cluster.vi"("error in (no error)"=w6692, "target cluster"=w6694, "Channel in"=w6690) -> ("error out"=w6693:errorcluster, "Channel out"=w6689:refnum<class "Channel.lvclass">)  [unwired: 7 in]
            n3070 = call-dynamic "Write target cluster.vi"("error in (no error)"=w6643, "target cluster"=w6644, "Channel in"=w6641) -> ("error out"=w6642:errorcluster, "Channel out"=w6640:refnum<class "Channel.lvclass">)  [unwired: 7 in]
            n3071 = call-dynamic "Write target cluster.vi"("error in (no error)"=w6590, "target cluster"=w6591, "Channel in"=w6588) -> ("error out"=w6589:errorcluster, "Channel out"=w6587:refnum<class "Channel.lvclass">)  [unwired: 7 in]
            n3072 = Flatten To String(anything=w6540, error in (no error)=w6538) -> (data string=w6579:string, error out=w6578:errorcluster)  [unwired: 2 in, 1 out]
            n3073 = Flatten To String(anything=w6694, error in (no error)=w6693) -> (data string=w6738:string, error out=w6737:errorcluster)  [unwired: 2 in, 1 out]
            n3074 = Flatten To String(anything=w6644, error in (no error)=w6642) -> (data string=w6678:string, error out=w6679:errorcluster)  [unwired: 2 in, 1 out]
            n3075 = Flatten To String(anything=w6591, error in (no error)=w6589) -> (data string=w6625:string, error out=w6626:errorcluster)  [unwired: 2 in, 1 out]
            n3076 = call "Write flatted cluster.vi"("error in (no error)"=w6578, "flatted cluster"=w6579, "Interface in"=w6542) -> ("error out"=w6575:errorcluster, "Interface out"=w6576:refnum<class "Interface.lvclass">)  [unwired: 7 in]
            n3077 = call "Write flatted cluster.vi"("error in (no error)"=w6737, "flatted cluster"=w6738, "Interface in"=w6696) -> ("error out"=w6734:errorcluster, "Interface out"=w6735:refnum<class "Interface.lvclass">)  [unwired: 7 in]
            n3078 = call "Write flatted cluster.vi"("error in (no error)"=w6679, "flatted cluster"=w6678, "Interface in"=w6645) -> ("error out"=w6682:errorcluster, "Interface out"=w6681:refnum<class "Interface.lvclass">)  [unwired: 7 in]
            n3079 = call "Write flatted cluster.vi"("error in (no error)"=w6626, "flatted cluster"=w6625, "Interface in"=w6592) -> ("error out"=w6629:errorcluster, "Interface out"=w6628:refnum<class "Interface.lvclass">)  [unwired: 7 in]
            n3080 = call-dynamic "Write Interface.vi"("error in (no error)"=w6734, "Interface.lvclass"=w6735, "Channel in"=w6689) -> ("error out"=w6732:errorcluster, "Channel out"=w6731:refnum<class "Channel.lvclass">)  [unwired: 7 in]
            n3081 = call-dynamic "Write Interface.vi"("error in (no error)"=w6575, "Interface.lvclass"=w6576, "Channel in"=w6537) -> ("error out"=w6573:errorcluster, "Channel out"=w6572:refnum<class "Channel.lvclass">)  [unwired: 7 in]
            n3082 = call-dynamic "Write Interface.vi"("error in (no error)"=w6682, "Interface.lvclass"=w6681, "Channel in"=w6640) -> ("error out"=w6684:errorcluster, "Channel out"=w6685:refnum<class "Channel.lvclass">)  [unwired: 7 in]
            n3083 = call-dynamic "Write Interface.vi"("error in (no error)"=w6629, "Interface.lvclass"=w6628, "Channel in"=w6587) -> ("error out"=w6631:errorcluster, "Channel out"=w6632:refnum<class "Channel.lvclass">)  [unwired: 7 in]
            n3084 = call "Write section_name.vi"("error in (no error)"=w6732, "section_name"="CCD_ACS1", "Channel in"=w6731) -> ("error out"=w6733:errorcluster, "Channel out"=w6728:refnum<class "Channel.lvclass">)  [unwired: 7 in]
            n3085 = call "Write section_name.vi"("error in (no error)"=w6573, "section_name"="CCD_ACS4", "Channel in"=w6572) -> ("error out"=w6574:errorcluster, "Channel out"=w6569:refnum<class "Channel.lvclass">)  [unwired: 7 in]
            n3086 = call "Write section_name.vi"("error in (no error)"=w6684, "section_name"="CCD_ACS2", "Channel in"=w6685) -> ("error out"=w6683:errorcluster, "Channel out"=w6688:refnum<class "Channel.lvclass">)  [unwired: 7 in]
            n3087 = call "Write section_name.vi"("error in (no error)"=w6631, "section_name"="CCD_ACS3", "Channel in"=w6632) -> ("error out"=w6630:errorcluster, "Channel out"=w6635:refnum<class "Channel.lvclass">)  [unwired: 7 in]
            n3088 = call-dynamic "save config.vi"("error in (no error)"=w6733, "file config"="lastsaved.cfg", "Channel in"=w6728) -> ("error out"=w6709:errorcluster, "Channel out"=w6708:refnum<class "Channel.lvclass">)  [unwired: 7 in]
            n3089 = call-dynamic "save config.vi"("error in (no error)"=w6574, "file config"="lastsaved.cfg", "Channel in"=w6569) -> ("error out"=w6555:errorcluster, "Channel out"=w6557:refnum<class "Channel.lvclass">)  [unwired: 7 in]
            n3090 = call-dynamic "save config.vi"("error in (no error)"=w6683, "file config"="lastsaved.cfg", "Channel in"=w6688) -> ("error out"=w6658:errorcluster, "Channel out"=w6661:refnum<class "Channel.lvclass">)  [unwired: 7 in]
            n3091 = local read "Filter2"() -> (w6657:u8)
            n3092 = local read "Filter4"() -> (w6554:u8)
            n3093 = call-dynamic "save config.vi"("error in (no error)"=w6630, "file config"="lastsaved.cfg", "Channel in"=w6635) -> ("error out"=w6605:errorcluster, "Channel out"=w6606:refnum<class "Channel.lvclass">)  [unwired: 7 in]
            n3094 = local read "Filter1"() -> (w6710:u8)
            n3095 = local read "Filter3"() -> (w6604:u8)
            n3096 = call-dynamic "Write Filter.vi"("error in (no error)"=w6658, "Filter"=w6657, "Channel in"=w6661) -> ("error out"=w6674:errorcluster, "Channel out"=w6660:refnum<class "Channel.lvclass">)  [unwired: 7 in]
            n3097 = call-dynamic "Write Filter.vi"("error in (no error)"=w6555, "Filter"=w6554, "Channel in"=w6557) -> ("error out"=w6568:errorcluster, "Channel out"=w6556:refnum<class "Channel.lvclass">)  [unwired: 7 in]
            n3098 = call-dynamic "Write Filter.vi"("error in (no error)"=w6709, "Filter"=w6710, "Channel in"=w6708) -> ("error out"=w6725:errorcluster, "Channel out"=w6724:refnum<class "Channel.lvclass">)  [unwired: 7 in]
            n3099 = call-dynamic "Write Filter.vi"("error in (no error)"=w6605, "Filter"=w6604, "Channel in"=w6606) -> ("error out"=w6607:errorcluster, "Channel out"=w6620:refnum<class "Channel.lvclass">)  [unwired: 7 in]
            n3100 = call-dynamic "Read Interface.vi"("error in (no error)"=w6674, "Channel in"=w6660) -> ("error out"=w6671:errorcluster, "Interface.lvclass"=w6670:refnum<class "Interface.lvclass">, "Channel out"=w6659:refnum<class "Channel.lvclass">)  [unwired: 7 in]
            n3101 = call-dynamic "Read Interface.vi"("error in (no error)"=w6725, "Channel in"=w6724) -> ("error out"=w6721:errorcluster, "Interface.lvclass"=w6720:refnum<class "Interface.lvclass">, "Channel out"=w6714:refnum<class "Channel.lvclass">)  [unwired: 7 in]
            n3102 = call-dynamic "Read Interface.vi"("error in (no error)"=w6568, "Channel in"=w6556) -> ("error out"=w6567:errorcluster, "Interface.lvclass"=w6566:refnum<class "Interface.lvclass">, "Channel out"=w6532:refnum<class "Channel.lvclass">)  [unwired: 7 in]
            n3103 = call-dynamic "Read Interface.vi"("error in (no error)"=w6607, "Channel in"=w6620) -> ("error out"=w6610:errorcluster, "Interface.lvclass"=w6611:refnum<class "Interface.lvclass">, "Channel out"=w6621:refnum<class "Channel.lvclass">)  [unwired: 7 in]
            n3104 = call-dynamic "Write Suffix.vi"("error in (no error)"=w6671, "Suffix"=w6743, "Interface in"=w6670) -> ("error out"=w6662:errorcluster, "Interface out"=w6665:refnum<class "Interface.lvclass">)  [unwired: 7 in]
            n3105 = call-dynamic "Write Suffix.vi"("error in (no error)"=w6721, "Suffix"=w6743, "Interface in"=w6720) -> ("error out"=w6711:errorcluster, "Interface out"=w6715:refnum<class "Interface.lvclass">)  [unwired: 7 in]
            n3106 = call-dynamic "Write Suffix.vi"("error in (no error)"=w6567, "Suffix"=w6743, "Interface in"=w6566) -> ("error out"=w6558:errorcluster, "Interface out"=w6561:refnum<class "Interface.lvclass">)  [unwired: 7 in]
            n3107 = call-dynamic "Write Suffix.vi"("error in (no error)"=w6610, "Suffix"=w6743, "Interface in"=w6611) -> ("error out"=w6619:errorcluster, "Interface out"=w6616:refnum<class "Interface.lvclass">)  [unwired: 7 in]
            n3108 = call-dynamic "Write ObsType.vi"("error in (no error)"=w6711, "ObsType"=w6742, "Interface in"=w6715) -> ("error out"=w6712:errorcluster, "Interface out"=w6716:refnum<class "Interface.lvclass">)  [unwired: 7 in]
            n3109 = call-dynamic "Write ObsType.vi"("error in (no error)"=w6662, "ObsType"=w6742, "Interface in"=w6665) -> ("error out"=w6663:errorcluster, "Interface out"=w6666:refnum<class "Interface.lvclass">)  [unwired: 7 in]
            n3110 = call-dynamic "Write ObsType.vi"("error in (no error)"=w6558, "ObsType"=w6742, "Interface in"=w6561) -> ("error out"=w6559:errorcluster, "Interface out"=w6562:refnum<class "Interface.lvclass">)  [unwired: 7 in]
            n3111 = call-dynamic "Write ObsType.vi"("error in (no error)"=w6619, "ObsType"=w6742, "Interface in"=w6616) -> ("error out"=w6618:errorcluster, "Interface out"=w6615:refnum<class "Interface.lvclass">)  [unwired: 7 in]
            n3112 = call-dynamic "Write Object.vi"("error in (no error)"=w6712, "Object"=w6746, "Interface in"=w6716) -> ("error out"=w6713:errorcluster, "Interface out"=w6717:refnum<class "Interface.lvclass">)  [unwired: 7 in]
